vi "Delete First and Last.vi"(11 "string in":string) -> (3 "string subset":string)   [LabVIEW 2020, in "Multi Error Cluster.lvlib"]
doc: "Deletes the first and last character of the string. Most commonly used to remove quotes from a JSON encoded field"
uses:
  <vilib>/MultiError/TokenizeJSON/Multi Error Cluster.lvlib
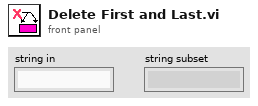
[diagram p1: front panel]
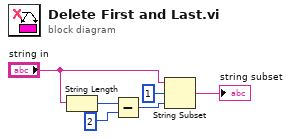
[diagram p0: block diagram]
diagram:
  n1 = String Length(string="string in") -> (length=w5:i32)
  n2 = Subtract(x=w5, y=2 ("offset (0)")) -> (x-y=w3:i32)
  n3 = String Subset(string="string in", offset (0)=1, length (rest)=w3) -> (substring=→"string subset":string)
